vi "Send_UART_msg.vi"(0 "VISA Refnum in":refnum<visa-resource-name>, 5 "Command":u8, 7 "Data 1":u8, 9 "Data 2":u8, 11 "error in (no error)":errorcluster) -> (4 "VISA Refnum out":refnum<visa-resource-name>, 8 "return count":u32, 15 "error out":errorcluster)   [LabVIEW 2015]
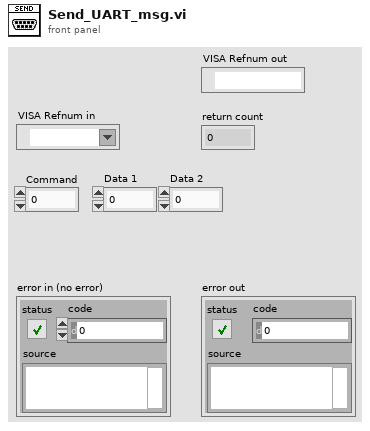
[diagram p1: front panel]
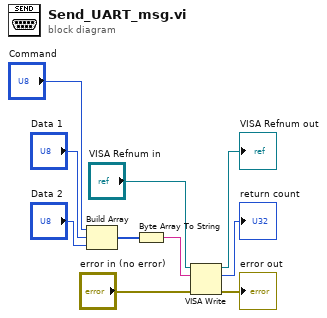
[diagram p0: block diagram]
diagram:
  n1 = Build Array("Command", "Data 1", "Data 2") -> (w1:u8[])
  n2 = Byte Array To String(unsigned byte array=w1) -> (string=w5:string)
  n3 = VISA Write(VISA resource name="VISA Refnum in", write buffer=w5, error in (no error)="error in (no error)") -> (VISA resource name out=→"VISA Refnum out":refnum<visa-resource-name>, return count=→"return count":u32, error out=→"error out":errorcluster)
